vi "sharp_ir_short.vi"(11 "ana_volts":dbl) -> (3 "eng_cm":dbl)   [LabVIEW 2013]
panel:
  in  "cm":dbl[](array[numeric])=[40.0, 40.0, 35.0, 30.0, 25.0, 20.0, 18.0, 16.0, 14.0, 12.0, 10.0, 9.0, 8.0, 7.0, 6.0, 5.0, 4.0, 3.0, 2.0, 0.0]
  in  "volts":dbl[](array[numeric])=[0.0, 0.35, 0.37, 0.41, 0.51, 0.63, 0.71, 0.805, 0.92, 1.03, 1.24, 1.4, 1.57, 1.77, 2.01, 2.37, 2.75, 3.0, 3.05, 5.0]
  # "This function is a transfer function for the Sharp IR GP2D120XJ00F short range IR rangefinder\nThis curve is copied directly from the Sharp spec sheet transfer curve. Units are cm in that sheet."
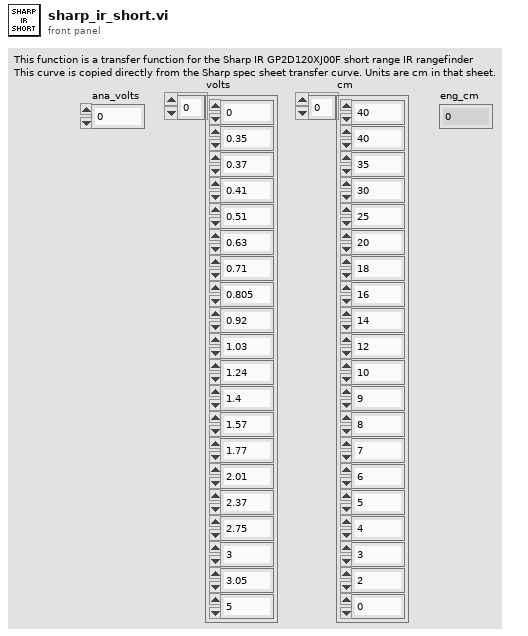
[diagram p1: front panel]
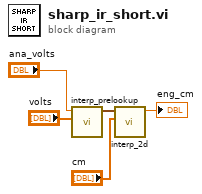
[diagram p0: block diagram]
diagram:
  n1 = call "interp_prelookup.vi"("x"="volts", "X"="ana_volts") -> ("prelookup"=w3:cluster{"frac":dbl, "num":u8})  [unwired: 8 in, 1 out]
  n2 = call "interp_2d.vi"("z"="cm", "prelookup"=w3) -> ("z"=→"eng_cm":dbl)  [unwired: 9 in]
